vi "NewAutoTrajectoryInterrupt.vi"(9 "command":string, 10 "commandtime":dbl, 11 "elapsedtime":dbl) -> ()   [LabVIEW 2023]
uses:
  <vilib>/Rock Robotics/WPI/ThirdParty/JAS_Junk/TrajLib/Trajectory_Library.lvlib
panel:
  # "mincemeat"
  # "potatoes"
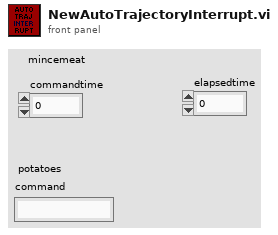
[diagram p1: front panel]
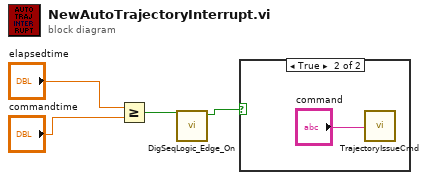
[diagram p0: block diagram]
diagram:
  n1 = Greater Or Equal?(x="elapsedtime", y="commandtime") -> (x >= y?=w1:bool)
  n2 = call <vilib>:"DigSeqLogic_Edge_On.vi"("Input"=w1) -> ("On Edge"=w2:bool)  [unwired: 10 in]
  n3 = case shown="True" w2 {
    frame False {
    }
    frame True {
      n4 = call "TrajectoryIssueCmd.vi"("Command"="command") -> ()  [unwired: 11 in]
    }
  }
